vi "writelog.vi"(7 "PDF path in":path, 8 "error in":errorcluster, 9 "data file path":path, 10 "Data table":string[][](table), 11 "Information":T1) -> (0 "error out":errorcluster)   [LabVIEW 2016]
uses:
  Controls/Information_tab_type.ctl
  <vilib>/Utility/file.llb/Write Delimited Spreadsheet (string).vi
panel:
  out "spreadsheet string":string
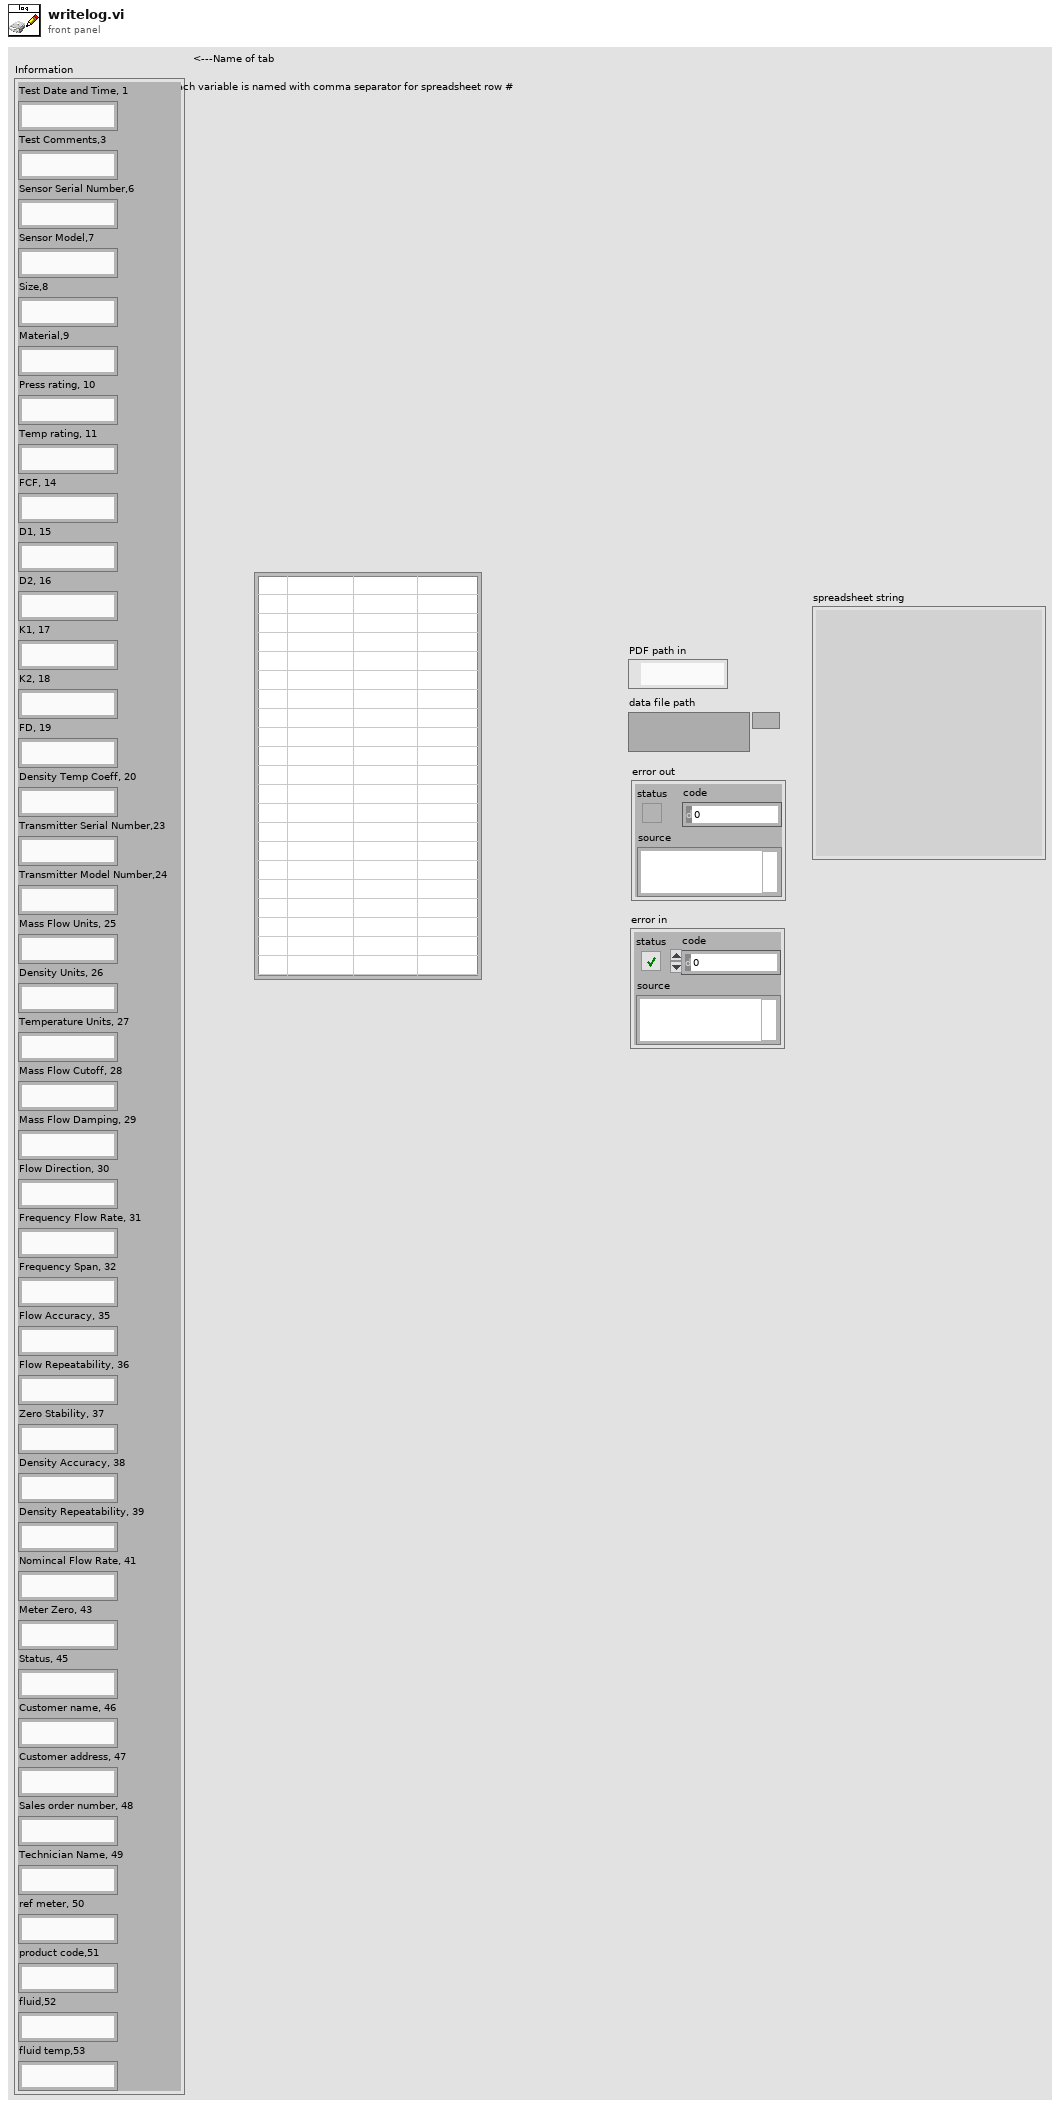
[diagram p1: front panel]
types:
  T1 = typedef "Information_tab_type.ctl" = cluster{"Test Date and Time, 1":string, "Test Comments,3":string, "Sensor Serial Number,6":string, "Sensor Model,7":string, "Size,8":string, "Material,9":string, "Press rating, 10":string, "Temp rating, 11":string, "FCF, 14":string, "D1, 15":string, "D2, 16":string, "K1, 17":string, "K2, 18":string, "FD, 19":string, "Density Temp Coeff, 20":string, "Transmitter Serial Number,23":string, "Transmitter Model Number,24":string, "Mass Flow Units, 25":string, "Density Units, 26":string, "Temperature Units, 27":string, "Mass Flow Cutoff, 28":string, "Mass Flow Damping, 29":string, "Flow Direction, 30":string, "Frequency Flow Rate, 31":string, "Frequency Span, 32":string, "Flow Accuracy, 35":string, "Flow Repeatability, 36":string, "Zero Stability, 37":string, "Density Accuracy, 38":string, "Density Repeatability, 39":string, "Nomincal Flow Rate, 41":string, "Meter Zero, 43":string, "Status, 45":string, "Customer name, 46":string, "Customer address, 47":string, "Sales order number, 48":string, "Technician Name, 49":string, "ref meter, 50":string, "product code,51":string, "fluid,52":string, "fluid temp,53":string}
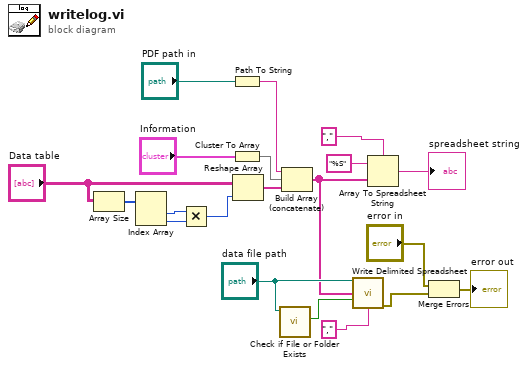
[diagram p0: block diagram]
diagram:
  n1 = Array Size(array="Data table") -> (size(s)=w19:i32[])
  n2 = Index Array(array=w19) -> (element #1=w18:i32, element #2=w17:i32)  [unwired: 2 in]
  n3 = Multiply(x=w18, y=w17) -> (x*y=w16:i32)
  n4 = Path To String(path="PDF path in") -> (string=w8:string)
  n5 = Cluster To Array(cluster="Information") -> (array=w14:string[])
  n6 = Reshape Array("Data table", w16) -> (w13:string[])
  n7 = call <vilib>:"Check if File or Folder Exists.vi"("path"="data file path") -> ("file or folder exists?"=w3:bool)  [unwired: 8 in, 2 out]
  n8 = Build Array (concatenate)(w8, w14, w13) -> (w2:string[])
  n9 = call-poly <vilib>:"Write Delimited Spreadsheet.vi"("file path (dialog if empty)"="data file path", "1D data"=w2, "append to file? (new file:F)"=w3, "delimiter (\\t)"="," ("delimiter (\\t)")) -> ("error out"=w1:errorcluster)  [unwired: 10 in, 1 out]
  n10 = Array To Spreadsheet String(delimiter (Tab)=",", array=w2, 3:"%S" ("format string")) -> (spreadsheet string=→"spreadsheet string":string)
  n11 = Merge Errors("error in", w1) -> (→"error out":errorcluster)
